vi "test moving avg.vi"() -> ()   [LabVIEW 2011]
panel:
  out "mean 3":dbl format="%0.2f"
  out "mean 2":dbl format="%0.2f"
  out "mean":dbl format="%0.2f"
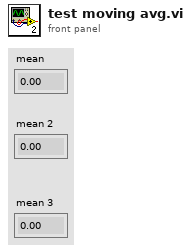
[diagram p1: front panel]
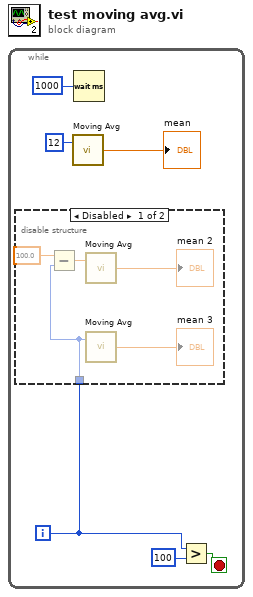
[diagram p0: block diagram]
diagram:
  n1 = while {
    i -> [w1]
    stop <- w6 stop-if-true
    n2 = disable-structure shown="Disabled" {
      disable-tunnel: w1 -> [w7 _]
      frame Disabled {
        n3 = Subtract(x=100.0, y=w7) -> (x-y=w9:dbl)
        n4 = call "Moving Avg.vi"("new measurement"=w9) -> ("mean"=→"mean 2":dbl)  [unwired: 1 in]
        n5 = call "Moving Avg.vi"("new measurement"=w7) -> ("mean"=→"mean 3":dbl)  [unwired: 1 in]
      }
      frame Enabled {
      }
    }
    n6 = call "Moving Avg.vi"("new measurement"=12) -> ("mean"=→"mean":dbl)  [unwired: 1 in]
    n7 = Wait (ms)(milliseconds to wait=u32 1000) -> ()  [unwired: 1 out]
    n8 = Greater?(x=w1, y=100) -> (0:w6:bool)
  }
